vi "Restart Spurious Emission Display Status.vi"(0 "VISA resource name":refnum<visa-resource-name>, 11 "error in (no error)":errorcluster) -> (4 "VISA resource name out":refnum<visa-resource-name>, 6 "Display Status":i32(ring) items=["Display"=1, "Not display"=0], 15 "error out":errorcluster)   [LabVIEW 2020, in "Anritsu Signal Analyzer Series.lvlib"]
doc: "Queries wheter the Spurious Emission Display Restart Status message is displayed on the trace."
uses:
  Anritsu Signal Analyzer Series.lvlib
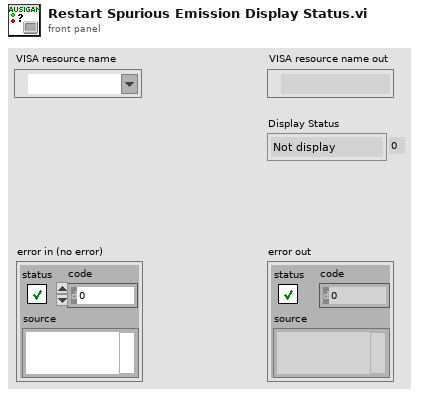
[diagram p1: front panel]
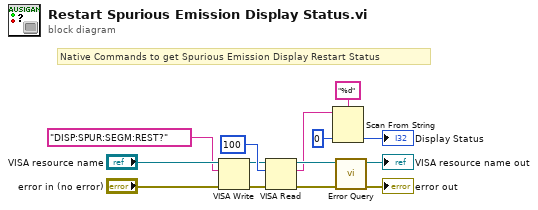
[diagram p0: block diagram]
diagram:
  # "Native Commands to get Spurious Emission Display Restart Status"
  n1 = VISA Write(VISA resource name="VISA resource name", write buffer="DISP:SPUR:SEGM:REST?" ("_Command"), error in (no error)="error in (no error)") -> (VISA resource name out=w7:refnum<visa-resource-name>, error out=w8:errorcluster)  [unwired: 1 out]
  n2 = VISA Read(VISA resource name=w7, byte count=u32 100 ("byte count (0)"), error in (no error)=w8) -> (VISA resource name out=w6:refnum<visa-resource-name>, read buffer=w2:string, error out=w5:errorcluster)  [unwired: 1 out]
  n3 = Scan From String(format string="%d" ("Format String"), input string=w2, default 1=0 ("_Default")) -> (output 1=→"Display Status":i32)  [unwired: 2 in, 3 out]
  n4 = call "Error Query.vi"("error in (no error)"=w5, "VISA resource name"=w6) -> ("error out"=→"error out":errorcluster, "VISA resource name out"=→"VISA resource name out":refnum<visa-resource-name>)  [unwired: 6 in, 2 out]
